vi "From Binary.vi"(8 "error in (no error)":errorcluster, 9 "byte order":T1(ring), 10 "Binary":string, 11 "Double Float in":refnum<class "AbsFunc_Two Term_DBL.lvclass">) -> (0 "error out":errorcluster, 2 "Remaning Binary":string, 3 "Double Float out":refnum<class "AbsFunc_Two Term_DBL.lvclass">)   [LabVIEW 2021, in "AbsFunc_Two Term_DBL.lvclass"]
uses:
  AbsFunc_Two Term_DBL.lvclass
  AbsFunc_Two Term_DBL.lvclass/AbsFunc_Two Term_DBL.ctl
  Abs_Types/Double Float/Abs_Double Float.lvclass
  Abs_Types/Numeric/Abs_Numeric.lvclass
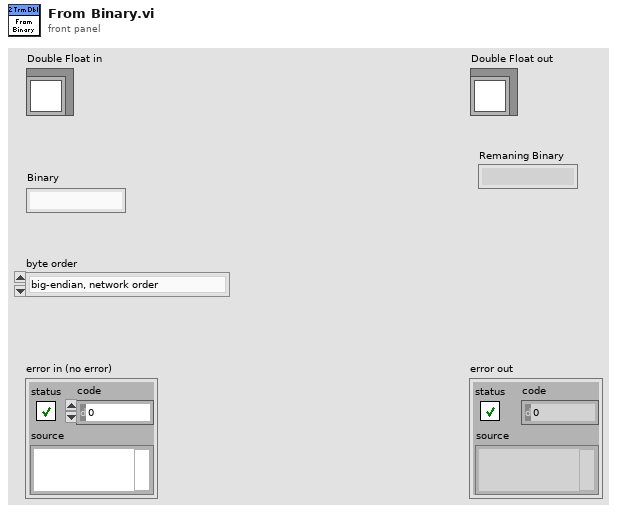
[diagram p1: front panel]
types:
  T1 = enum16{"big-endian, network order", "native, host order", "little-endian"}
  T2 = typedef "AbsFunc_Two Term DBL.lvclass/Abstract Type.ctl" = refnum<class "Abs_Double Float.lvclass">
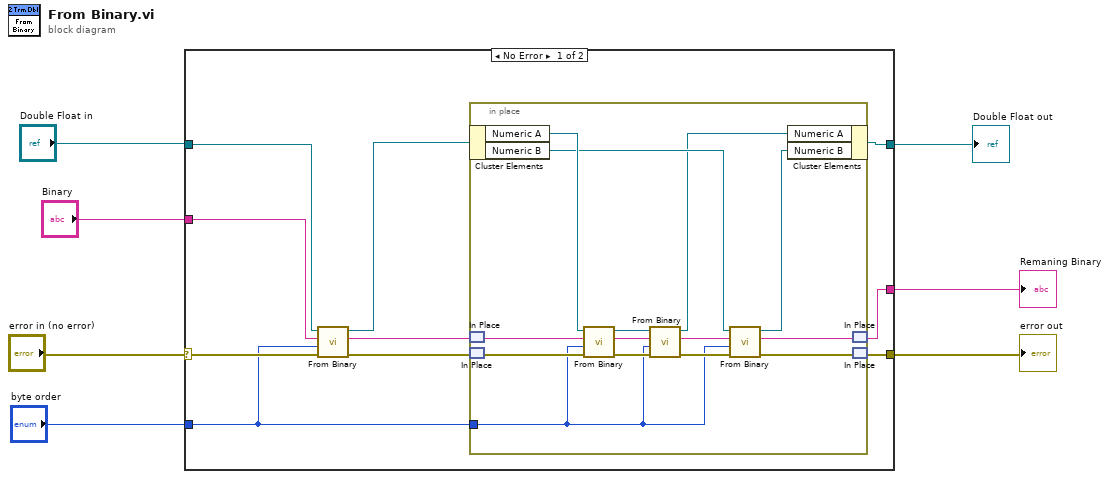
[diagram p0: block diagram]
diagram:
  n1 = case shown="No Error" "error in (no error)" {
    selector: "error in (no error)" -> [w15 w33]
    tunnel: "Binary" -> [w11 w34]
    tunnel: [w17 w33] -> w3
    tunnel: "byte order" -> [w14 _]
    tunnel: [w16 w34] -> w4
    tunnel: "Double Float in" -> [w13 w32]
    tunnel: [w8 w32] -> w1
    frame No Error {
      n2 = call-parent "From Binary.vi"("error in (no error)"=w15, "byte order"=w14, "Binary"=w11, "Double Float in"=w13) -> ("error out"=w12:errorcluster, "Remaning Binary"=w10:string, "Double Float out"=w9:refnum<class "AbsFunc_Two Term_DBL.lvclass">)  [unwired: 5 in]
      n3 = in-place {
        in-place-border: w14 -> [w18]
        n4 = in-place-cluster #1(w9) -> ("Numeric A"=w31:T2, "Numeric B"=w26:refnum<class "Abs_Numeric.lvclass">)
        n5 = in-place-match #2(w10) -> (w29:string)
        n6 = in-place-match #3(w12) -> (w30:errorcluster)
        n7 = call-dynamic "From Binary.vi"("error in (no error)"=w30, "byte order"=w18, "Binary"=w29, "Double Float in"=w31) -> ("error out"=w24:errorcluster, "Remaning Binary"=w22:string, "Double Float out"=w23:T2)  [unwired: 5 in]
        n8 = call-dynamic "From Binary.vi"("error in (no error)"=w24, "byte order"=w18, "Binary"=w22, "Double Float in"=w23) -> ("error out"=w19:errorcluster, "Remaning Binary"=w20:string, "Double Float out"=w21:T2)  [unwired: 5 in]
        n9 = call-dynamic "From Binary.vi"("error in (no error)"=w19, "byte order"=w18, "Binary"=w20, "Type in"=w26) -> ("error out"=w28:errorcluster, "Remaning Binary"=w27:string, "Type out"=w25:refnum<class "Abs_Numeric.lvclass">)  [unwired: 5 in]
        n10 = in-place-cluster #1("Numeric A"=w21, "Numeric B"=w25) -> (w8:refnum<class "AbsFunc_Two Term_DBL.lvclass">)
        n11 = in-place-match #2(w27) -> (w16:string)
        n12 = in-place-match #3(w28) -> (w17:errorcluster)
      }
    }
    frame Error {
    }
  }
  "error out" <- w3
  "Double Float out" <- w1
  "Remaning Binary" <- w4
